vi "JSON RPC Server (test).vi"() -> ()   [LabVIEW 2020]
uses:
  Lib/JSON-RPC/Classes/Server/Add Response (Result from Request).vi
  Lib/JSON-RPC/Classes/Server/Add Response (Server Error from Request).vi
  Lib/JSON-RPC/Classes/Server/Add Response (Internal Error from Request).vi
  Lib/JSON-RPC/Classes/Server/Send Request (Sync).vi
  Lib/JSON-RPC/Classes/Server/JSONRPC Server.lvclass
panel:
  out "header":string
  out "request":string
  out "response":string
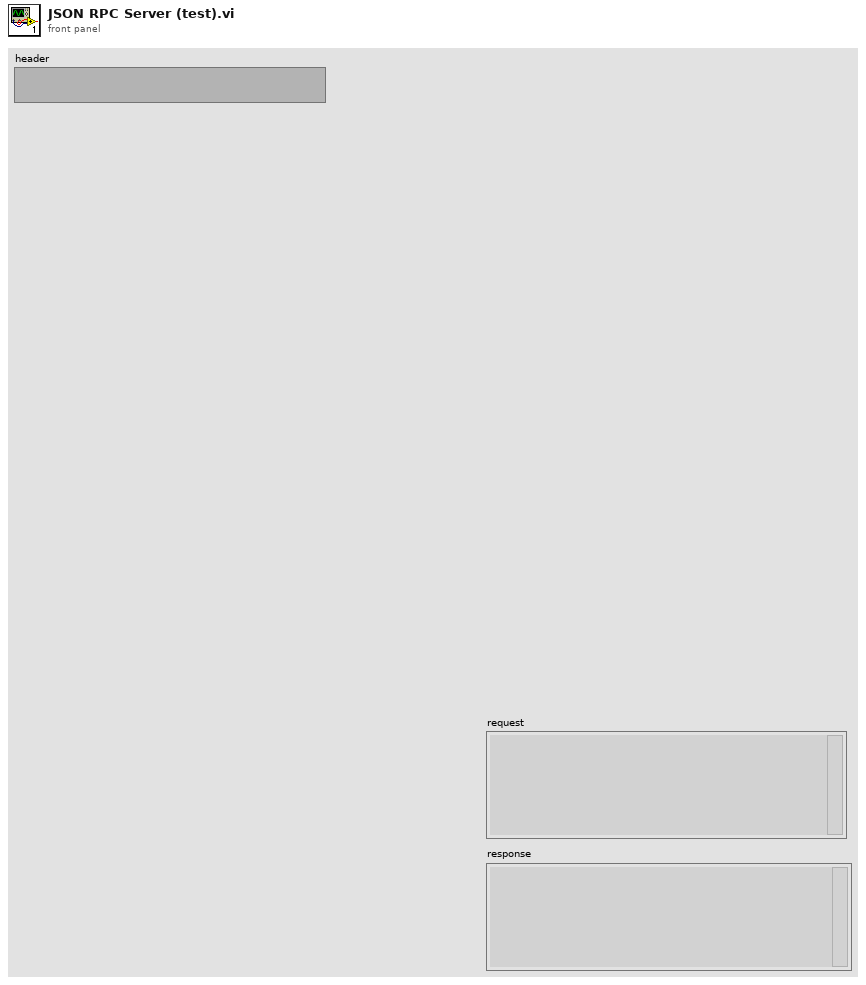
[diagram p1: front panel]
types:
  T1 = enum16{"Standard", "Buffered", "CRLF", "Immediate"}
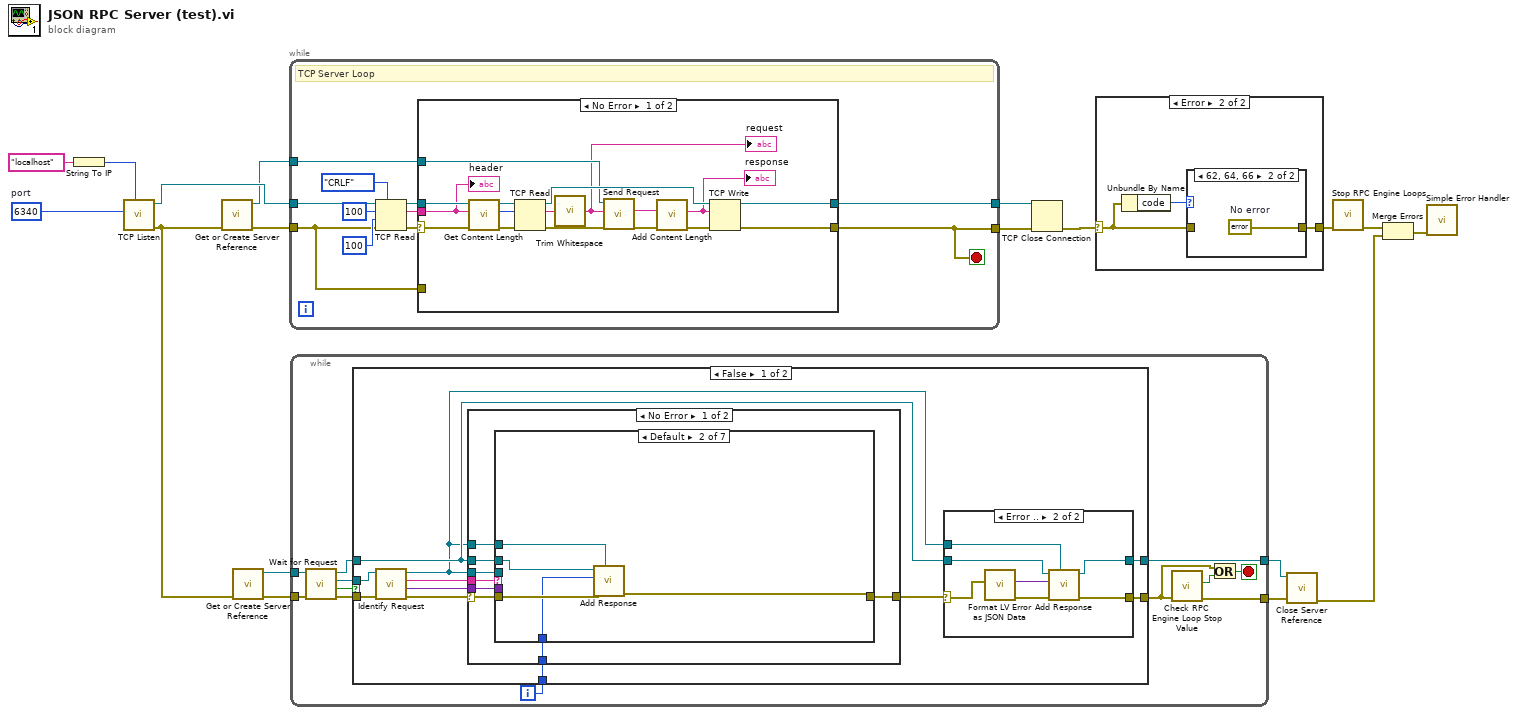
[diagram p0: block diagram]
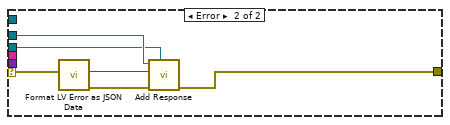
[diagram p9: hidden frame]
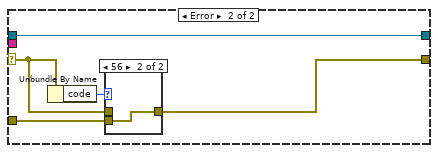
[diagram p13: hidden frame]
diagram:
  w16 = u16 6340  # port
  n1 = String To IP(1:"localhost" ("name")) -> (0:w15:u32)
  n2 = call <vilib>:"TCP Listen.vi"("net address"=w15, "port"=w16) -> ("error out"=w3:errorcluster, "connection ID"=w12:refnum<k5>)  [unwired: 5 in, 3 out]
  n3 = call "Get or Create Server Reference.vi"("error in (no error)"=w3) -> ("error out"=w11:errorcluster, "Server Out"=w10:refnum<class "JSONRPC Server.lvclass">)  [unwired: 9 in]
  n4 = call "Get or Create Server Reference.vi"("error in (no error)"=w3) -> ("error out"=w8:errorcluster, "Server Out"=w1:refnum<class "JSONRPC Server.lvclass">)  [unwired: 9 in]
  n5 = while {
    tunnel: [w19] -> w17
    tunnel: [w26] -> w18
    tunnel: w12 -> [w22]
    tunnel: w11 -> [w23]
    tunnel: w10 -> [w20]
    stop <- w19 stop-if-true
    # "TCP Server Loop"
    n6 = TCP Read(connection ID=w22, bytes to read=100, error in (no error)=w23, 7:T1."CRLF" ("mode (standard)"), 9:100 ("timeout ms (25000)")) -> (connection ID out=w27:refnum<k5>, data out=w21:string, error out=w25:errorcluster)
    n7 = case shown="No Error" w25 {
      selector: w25 -> [w45 w49]
      tunnel: [w39 w47] -> w19
      tunnel: w23 -> [_ w48]
      tunnel: [w40 w46] -> w26
      tunnel: w27 -> [w43 w46]
      tunnel: w21 -> [w42 _]
      tunnel: w20 -> [w36 _]
      frame No Error {
        n8 = call "Get Content Length.vi"("error in (no error)"=w45, "header"=w42) -> ("error out"=w44:errorcluster, "content length"=w41:i32)  [unwired: 8 in]
        n9 = TCP Read(connection ID=w43, bytes to read=w41, error in (no error)=w44) -> (connection ID out=w38:refnum<k5>, data out=w31:string, error out=w37:errorcluster)  [unwired: 2 out]
        n10 = call <vilib>:"Trim Whitespace.vi"("string"=w31) -> ("trimmed string"=w30:string)  [unwired: 1 in]
        "request" <- w30
        n11 = call-poly "Send Request.vi"("error in (no error)"=w37, "JSON Request String"=w30, "JSONRPC Server in"=w36) -> ("error out"=w35:errorcluster, "JSON Response String"=w32:string)  [unwired: 6 in, 1 out]
        n12 = call "Add Content Length.vi"("error in (no error)"=w35, "JSON Response String in"=w32) -> ("error out"=w34:errorcluster, "JSON Response String out"=w33:string)  [unwired: 8 in]
        "response" <- w33
        n13 = TCP Write(connection ID=w38, data in=w33, error in (no error)=w34) -> (connection ID out=w40:refnum<k5>, error out=w39:errorcluster)  [unwired: 1 in, 1 out]
        "header" <- w42
      }
      frame Error {
        n14 = Unbundle By Name(w49) -> ("code"=w50:i32)
        n15 = case shown="56" w50 {
          tunnel: w49 -> [w51 _]
          tunnel: w48 -> [_ w52]
          tunnel: [w51 w52] -> w47
          frame Default {
          }
          frame 56 {
          }
        }
      }
    }
  }
  n16 = while {
    tunnel: w8 -> [w64]
    tunnel: w1 -> [w63]
    tunnel: [w58] -> w7
    tunnel: [w57] -> w6
    i -> [w53]
    stop <- w54 stop-if-true
    n17 = call "Wait for Request.vi"("error in (no error)"=w64, "Server in"=w63) -> ("error out"=w62:errorcluster, "timed out?"=w59:bool, "Request"=w61:refnum<class "Request.lvclass">, "Server out"=w60:refnum<class "JSONRPC Server.lvclass">)  [unwired: 6 in]
    n18 = case shown="False" w59 {
      tunnel: w62 -> [w69 w111]
      tunnel: w61 -> [w75 _]
      tunnel: w60 -> [w67 w110]
      tunnel: [w72 w111] -> w55
      tunnel: [w71 w110] -> w57
      tunnel: w53 -> [w65 _]
      frame False {
        n19 = call "Identify Request.vi"("error in (no error)"=w69, "Request in"=w75) -> ("error out"=w70:errorcluster, "params"=w74:variant, "method"=w68:string, "Request out"=w66:refnum<class "Request.lvclass">)  [unwired: 5 in, 1 out]
        n20 = case shown="No Error" w70 {
          selector: w70 -> [w90 w109]
          tunnel: w74 -> [w87 _]
          tunnel: w67 -> [w92 w107]
          tunnel: w66 -> [w91 w106]
          tunnel: [w89 w104] -> w73
          tunnel: w68 -> [w88 _]
          tunnel: w66 -> [w86 _]
          tunnel: w65 -> [w85 _]
          frame No Error {
            n21 = case shown="Default" w88 {
              tunnel: w92 -> [_ w97 _ _ _ _ _]
              tunnel: w91 -> [_ _ _ _ _ _ _]
              tunnel: w90 -> [w93 w98 w99 w100 w101 w102 w103]
              tunnel: [w93 w94 w99 w100 w101 w102 w103] -> w89
              tunnel: w87 -> [_ _ _ _ _ _ _]
              tunnel: w86 -> [_ w96 _ _ _ _ _]
              tunnel: w85 -> [_ w95 _ _ _ _ _]
              frame "rpc_server_init" {
              }
              frame Default {
                n22 = call-poly "Add Response.vi"("Request"=w96, "error in (no error)"=w98, "JSON Value in"=w95, "Server in"=w97) -> ("error out"=w94:errorcluster)  [unwired: 5 in, 2 out]
              }
              frame "rpc_server_dispatch" {
              }
              frame "rpc_server_launch_module" {
              }
              frame "rpc_server_shutdown_module" {
              }
              frame "rpc_server_broadcast" {
              }
              frame "rpc_server_shutdown" {
              }
            }
          }
          frame Error {
            n23 = call "Format LV Error as JSON Data.vi"("error in"=w109) -> ("error out"=w108:errorcluster, "Error Value out"=w105:variant)  [unwired: 9 in]
            n24 = call-poly "Add Response.vi"("Request"=w106, "error in (no error)"=w108, "data"=w105, "Server in"=w107) -> ("error out"=w104:errorcluster)  [unwired: 5 in, 2 out]
          }
        }
        n25 = case shown="Error .." w73 {
          selector: w73 -> [w77 w82]
          tunnel: [w77 w81] -> w72
          tunnel: w67 -> [w76 w79]
          tunnel: [w76 w80] -> w71
          tunnel: w66 -> [_ w78]
          frame No Error {
          }
          frame Error {
            n26 = call "Format LV Error as JSON Data.vi"("error in"=w82) -> ("error out"=w84:errorcluster, "Error Value out"=w83:variant)  [unwired: 9 in]
            n27 = call-poly "Add Response.vi"("Request"=w78, "error in (no error)"=w84, "data"=w83, "Server in"=w79) -> ("error out"=w81:errorcluster, "Server out"=w80:refnum<class "JSONRPC Server.lvclass">)  [unwired: 5 in, 1 out]
          }
        }
      }
      frame True {
      }
    }
    n28 = call "Check RPC Engine Loop Stop Value.vi"("error in (no error)"=w55) -> ("error out"=w58:errorcluster, "stopped?"=w56:bool)  [unwired: 9 in]
    n29 = Or(x=w55, y=w56) -> (x .or. y?=w54:bool)
  }
  n30 = TCP Close Connection(connection ID=w18, error in (no error)=w17) -> (error out=w14:errorcluster)  [unwired: 2 out]
  n31 = case shown="Error" w14 {
    selector: w14 -> [w112 w114]
    tunnel: [w112 w113] -> w9
    frame No Error {
    }
    frame Error {
      n32 = Unbundle By Name(w114) -> ("code"=w115:i32)
      n33 = case shown="62, 64, 66" w115 {
        tunnel: w114 -> [w116 _]
        tunnel: [w116 w117] -> w113
        frame Default {
        }
        frame 62, 64, 66 {
          w117 = errorcluster {"status"=FALSE, "code"=0, "source"=""}  # No error
        }
      }
    }
  }
  n34 = call "Close Server Reference.vi"("error in (no error)"=w7, "Server in"=w6) -> ("error out"=w2:errorcluster)  [unwired: 9 in]
  n35 = call "Stop RPC Engine Loops.vi"("error in (no error)"=w9) -> ("error out"=w5:errorcluster)  [unwired: 10 in]
  n36 = Merge Errors(w5, w2) -> (w4:errorcluster)
  n37 = call <vilib>:"Simple Error Handler.vi"("error in (no error)"=w4) -> ()  [unwired: 1 in, 8 out]
